vi "write byte array.vi"(8 "error in":errorcluster, 10 "specs":T1[](array[typedef]), 11 "message":variant) -> (0 "error out":errorcluster, 3 "byte array":u8[](array[numeric]))   [LabVIEW 2013, in "protocol buffers encoder.lvlib"]
uses:
  protocol buffers encoder.lvlib
  message specification.ctl
  field descriptor.ctl
  quantity.ctl
  wire type.ctl
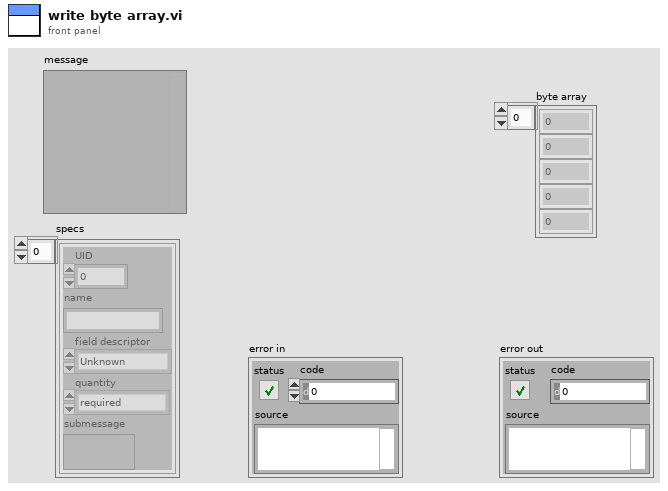
[diagram p1: front panel]
types:
  T1 = typedef "protocol buffers encoder.lvlib/message specification.ctl" = cluster{"UID":u64, "name":string, "field descriptor":T2, "quantity":T3, "submessage":variant}
  T2 = typedef "protocol buffers encoder.lvlib/field descriptor.ctl" = enum16{"Unknown", "dbl", "sgl", "i64", "u64", "i32", "fixed64", "fixed32", "bool", "string", "group", "message", "bytes", "u32", "enum", "sfixed32", "sfixed64", "sint32", "sint64"}
  T3 = typedef "protocol buffers encoder.lvlib/quantity.ctl" = enum16{"required", "optional", "repeated", "repeated/packed"}
  T4 = typedef "protocol buffers encoder.lvlib/wire type.ctl" = enum8{"Varint", "64 bit", "Length Delimited", "Start Group", "End Group", "32 bit"}
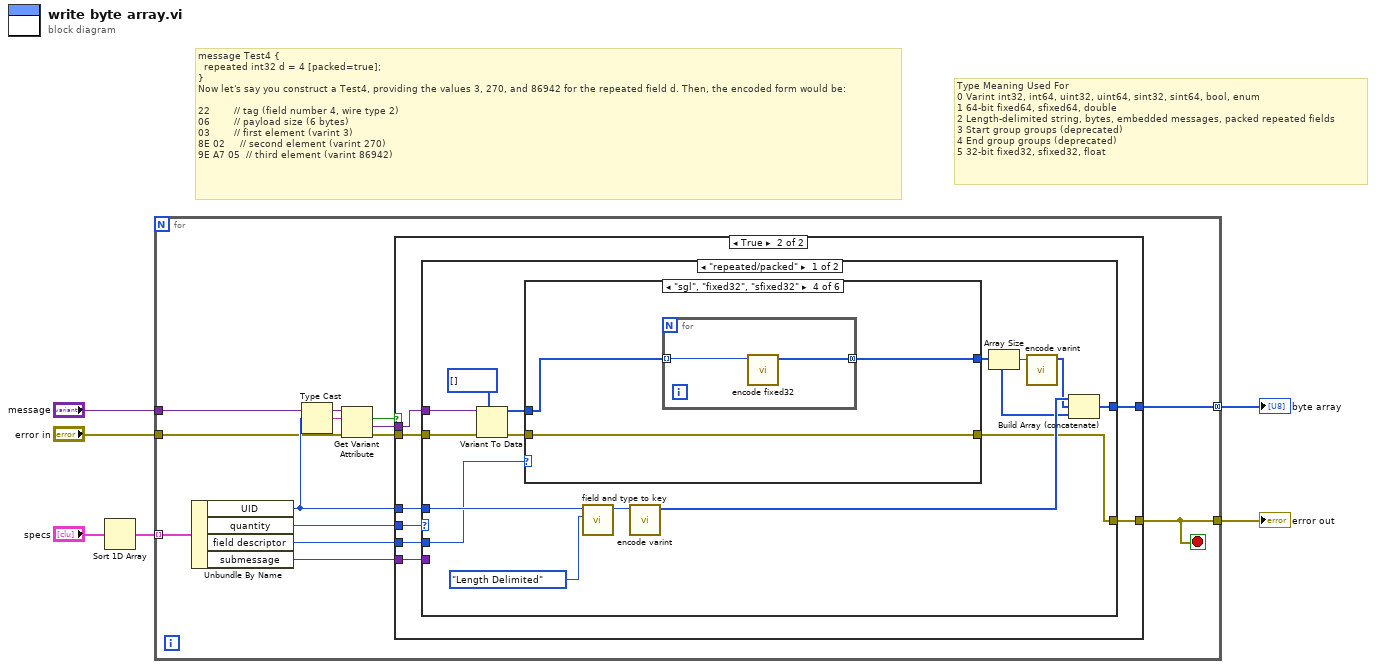
[diagram p0: block diagram]
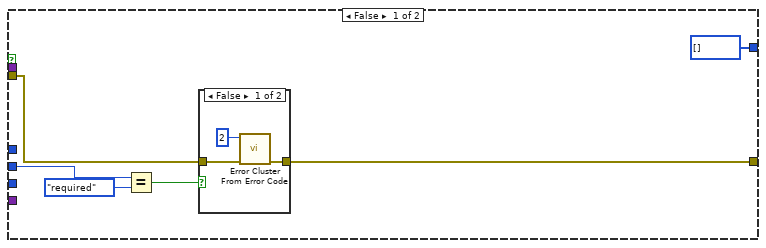
[diagram p2: hidden frame]
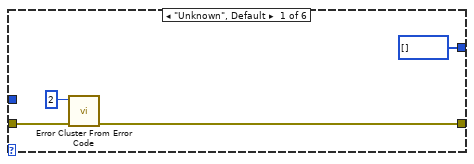
[diagram p4: hidden frame]
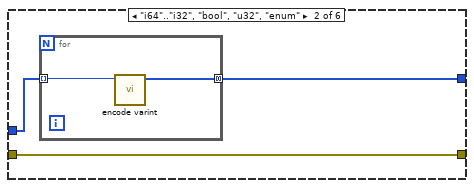
[diagram p5: hidden frame]
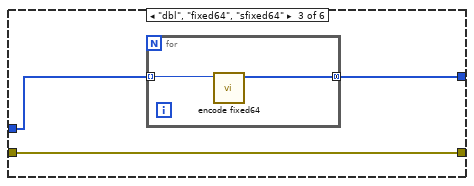
[diagram p6: hidden frame]
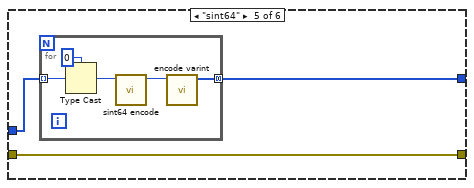
[diagram p7: hidden frame]
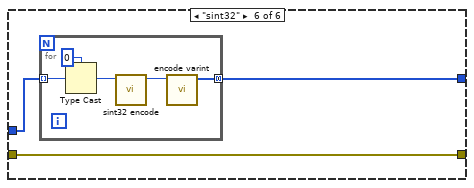
[diagram p8: hidden frame]
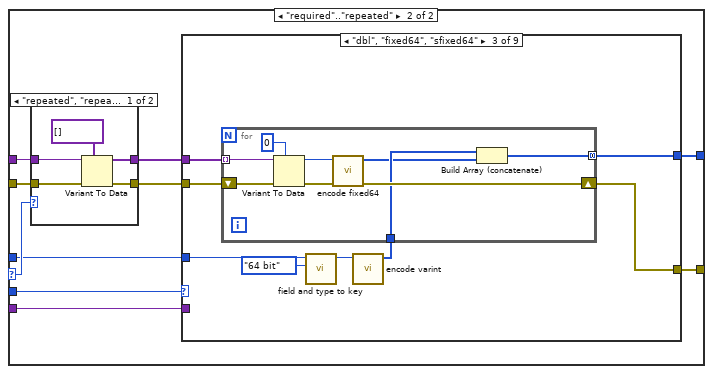
[diagram p9: hidden frame]
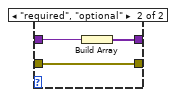
[diagram p10: hidden frame]
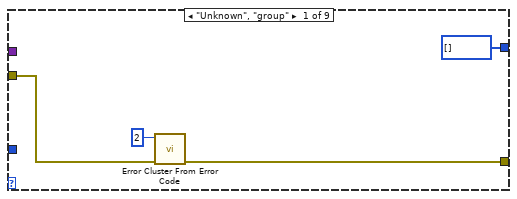
[diagram p11: hidden frame]
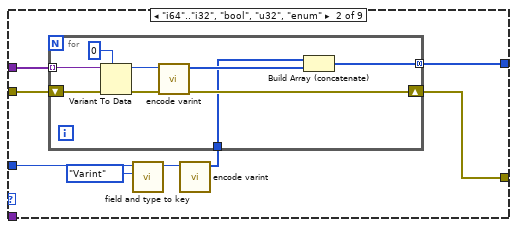
[diagram p12: hidden frame]
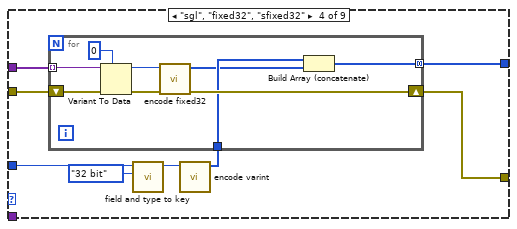
[diagram p13: hidden frame]
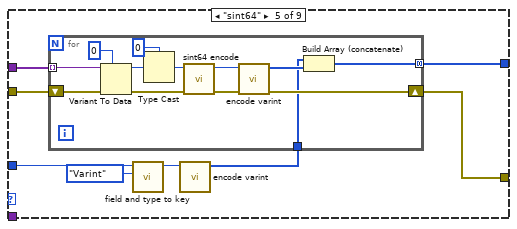
[diagram p14: hidden frame]
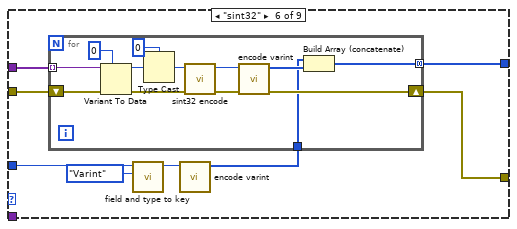
[diagram p15: hidden frame]
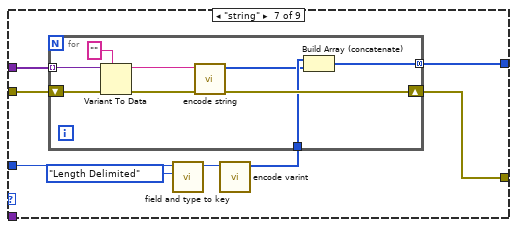
[diagram p16: hidden frame]
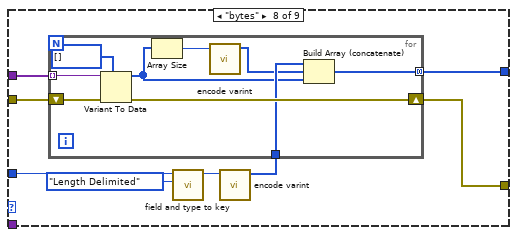
[diagram p17: hidden frame]
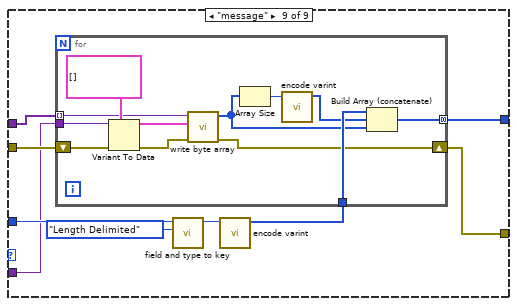
[diagram p18: hidden frame]
diagram:
  # "message Test4 {\n  repeated int32 d = 4 [packed=true];\n}\nNow let's say you construct a Test4, providing the values 3, 270, and 86942 for the repeated field d. Then, the encoded form would be:\n\n22        // tag (field number 4, wire type 2)\n06        // payload size (6 bytes)\n03        // first element (varint 3)\n8E 02     // second element (varint 270)\n9E A7 05  // third element (varint 86942)"
  # "Type\tMeaning\tUsed For\n0\tVarint\tint32, int64, uint32, uint64, sint32, sint64, bool, enum\n1\t64-bit\tfixed64, sfixed64, double\n2\tLength-delimited\tstring, bytes, embedded messages, packed repeated fields\n3\tStart group\tgroups (deprecated)\n4\tEnd group\tgroups (deprecated)\n5\t32-bit\tfixed32, sfixed32, float"
  n1 = Sort 1D Array(array="specs") -> (sorted array=w3:T1[])
  n2 = for {
    tunnel: w3 -> [w19] mode=indexing
    tunnel: "message" -> [w18]
    tunnel: [w13] -> w4
    tunnel: [w8] -> w2 mode=concatenating
    tunnel: "error in" -> [w7]
    stop <- w13 stop-if-true
    n3 = Unbundle By Name(w19) -> ("UID"=w9:u64, "quantity"=w10:T3, "field descriptor"=w12:T2, "submessage"=w11:variant)
    n4 = Type Cast(x=w9) -> (*(type *) &x=w17:string)  [unwired: 1 in]
    n5 = Get Variant Attribute(Variant=w18, name=w17, error in=w7) -> (found=w14:bool, value=w15:variant, error out=w16:errorcluster)  [unwired: 1 in, 1 out]
    n6 = case shown="True" w14 {
      tunnel: w16 -> [w22 w35]
      tunnel: w15 -> [_ w34]
      tunnel: w10 -> [w25 w32]
      tunnel: [w21 w36] -> w13
      tunnel: w12 -> [_ w37]
      tunnel: w11 -> [_ w33]
      tunnel: w9 -> [_ w31]
      tunnel: [u8[] [] w30] -> w8
      frame False {
        n7 = Equal?(x=w25, y=quantity."required") -> (x = y?=w23:bool)
        n8 = case shown="False" w23 {
          tunnel: w22 -> [w27 w29]
          tunnel: [w26 w29] -> w21
          frame False {
            n9 = call <vilib>:"Error Cluster From Error Code.vi"("error in (no error)"=w27, "error code (0)"=2) -> ("error out"=w26:errorcluster)  [unwired: 7 in]
          }
          frame True {
          }
        }
      }
      frame True {
        n10 = case shown="\"repeated/packed\"" w32 {
          selector: w32 -> [_ w90]
          tunnel: w37 -> [w44 w97]
          tunnel: [w42 w96] -> w36
          tunnel: w35 -> [w50 w95]
          tunnel: w34 -> [w51 w94]
          tunnel: w33 -> [_ w91]
          tunnel: w31 -> [w47 w89]
          tunnel: [w45 w88] -> w30
          frame "repeated/packed" {
            n11 = Variant To Data(error in=w50, type=u64[] [], Variant=w51) -> (data=w41:u64[], error out=w43:errorcluster)
            n12 = case shown="\"sgl\", \"fixed32\", \"sfixed32\"" w44 {
              tunnel: w43 -> [w55 w59 w64 w69 w74 w82]
              tunnel: [w54 w59 w64 w69 w74 w82] -> w42
              tunnel: w41 -> [_ w58 w63 w68 w73 w81]
              tunnel: [u8[] [] ("byte array out") w57 w62 w67 w72 w80] -> w38
              frame "Unknown", Default {
                n13 = call <vilib>:"Error Cluster From Error Code.vi"("error in (no error)"=w55, "error code (0)"=2) -> ("error out"=w54:errorcluster)  [unwired: 7 in]
              }
              frame "i64".."i32", "bool", "u32", "enum" {
                n14 = for {
                  tunnel: w58 -> [w61] mode=indexing
                  tunnel: [w60] -> w57 mode=concatenating
                  n15 = call "encode varint.vi"("value"=w61) -> ("byte array out"=w60:u8[])  [unwired: 10 in]
                }
              }
              frame "dbl", "fixed64", "sfixed64" {
                n16 = for {
                  tunnel: w63 -> [w66] mode=indexing
                  tunnel: [w65] -> w62 mode=concatenating
                  n17 = call "encode fixed64.vi"("U64"=w66) -> ("byte array out"=w65:u8[])  [unwired: 10 in]
                }
              }
              frame "sgl", "fixed32", "sfixed32" {
                n18 = for {
                  tunnel: w68 -> [w70] mode=indexing
                  tunnel: [w71] -> w67 mode=concatenating
                  n19 = call "encode fixed32.vi"("u32"=w70) -> ("byte array out"=w71:u8[])  [unwired: 10 in]
                }
              }
              frame "sint64" {
                n20 = for {
                  tunnel: w73 -> [w78] mode=indexing
                  tunnel: [w79] -> w72 mode=concatenating
                  n21 = Type Cast(type=i64 0, x=w78) -> (*(type *) &x=w76:i64)
                  n22 = call "sint64 encode.vi"("sint64"=w76) -> ("zigzag32"=w77:u64)  [unwired: 10 in]
                  n23 = call "encode varint.vi"("value"=w77) -> ("byte array out"=w79:u8[])  [unwired: 10 in]
                }
              }
              frame "sint32" {
                n24 = for {
                  tunnel: w81 -> [w86] mode=indexing
                  tunnel: [w87] -> w80 mode=concatenating
                  n25 = Type Cast(type=0, x=w86) -> (*(type *) &x=w84:i32)
                  n26 = call "sint32 encode.vi"("sint32"=w84) -> ("zigzag32"=w83:u32)  [unwired: 10 in]
                  n27 = call "encode varint.vi"("value"=w83) -> ("byte array out"=w87:u8[])  [unwired: 10 in]
                }
              }
            }
            n28 = call "field and type to key.vi"("wire type"=wire_type."Length Delimited", "field number"=w47) -> ("key"=w49:u64)  [unwired: 9 in]
            n29 = call "encode varint.vi"("value"=w49) -> ("byte array out"=w46:u8[])  [unwired: 10 in]
            n30 = Array Size(array=w38) -> (size(s)=w39:i32)
            n31 = call "encode varint.vi"("value"=w39) -> ("byte array out"=w40:u8[])  [unwired: 10 in]
            n32 = Build Array (concatenate)(w46, w40, w38) -> (w45:u8[])
          }
          frame "required".."repeated" {
            n33 = case shown="\"repeated\", \"repeated/packed\"" w90 {
              tunnel: w95 -> [w100 w103]
              tunnel: w94 -> [w101 w105]
              tunnel: [w99 w104] -> w93
              tunnel: [w98 w103] -> w92
              frame "repeated", "repeated/packed" {
                n34 = Variant To Data(error in=w100, type=variant[] [], Variant=w101) -> (data=w99:variant[], error out=w98:errorcluster)
              }
              frame "required", "optional" {
                n35 = Build Array(w105) -> (w104:variant[])
              }
            }
            n36 = case shown="\"dbl\", \"fixed64\", \"sfixed64\"" w97 {
              tunnel: [w108 w115 w131 w147 w163 w182 w201 w217 w235] -> w96
              tunnel: w93 -> [_ w116 w132 w148 w164 w183 w202 w218 w236]
              tunnel: w92 -> [w106 w117 w133 w149 w165 w184 w203 w219 w237]
              tunnel: w91 -> [_ _ _ _ _ _ _ _ w229]
              tunnel: w89 -> [_ w113 w129 w145 w161 w180 w199 w215 w233]
              tunnel: [u8[] [] w110 w126 w142 w158 w177 w196 w212 w230] -> w88
              frame "Unknown", "group" {
                n37 = call <vilib>:"Error Cluster From Error Code.vi"("error in (no error)"=w106, "error code (0)"=2) -> ("error out"=w108:errorcluster)  [unwired: 7 in]
              }
              frame "i64".."i32", "bool", "u32", "enum" {
                n38 = call "field and type to key.vi"("wire type"=wire_type."Varint", "field number"=w113) -> ("key"=w114:u64)  [unwired: 9 in]
                n39 = call "encode varint.vi"("value"=w114) -> ("byte array out"=w111:u8[])  [unwired: 10 in]
                n40 = for {
                  shift-right: [w122] -> w115
                  shift-left: w117 -> [w124]
                  tunnel: w116 -> [w125] mode=indexing
                  tunnel: w111 -> [w120]
                  tunnel: [w118] -> w110 mode=concatenating
                  n41 = Variant To Data(error in=w124, type=u64 0, Variant=w125) -> (data=w119:u64, error out=w122:errorcluster)
                  n42 = call "encode varint.vi"("value"=w119) -> ("byte array out"=w121:u8[])  [unwired: 10 in]
                  n43 = Build Array (concatenate)(w120, w121) -> (w118:u8[])
                }
              }
              frame "dbl", "fixed64", "sfixed64" {
                n44 = call "field and type to key.vi"("wire type"=wire_type."64 bit", "field number"=w129) -> ("key"=w130:u64)  [unwired: 9 in]
                n45 = call "encode varint.vi"("value"=w130) -> ("byte array out"=w127:u8[])  [unwired: 10 in]
                n46 = for {
                  shift-right: [w138] -> w131
                  shift-left: w133 -> [w140]
                  tunnel: w132 -> [w141] mode=indexing
                  tunnel: w127 -> [w137]
                  tunnel: [w136] -> w126 mode=concatenating
                  n47 = Variant To Data(error in=w140, type=u64 0, Variant=w141) -> (data=w135:u64, error out=w138:errorcluster)
                  n48 = call "encode fixed64.vi"("U64"=w135) -> ("byte array out"=w134:u8[])  [unwired: 10 in]
                  n49 = Build Array (concatenate)(w137, w134) -> (w136:u8[])
                }
              }
              frame "sgl", "fixed32", "sfixed32" {
                n50 = call "field and type to key.vi"("wire type"=wire_type."32 bit", "field number"=w145) -> ("key"=w146:u64)  [unwired: 9 in]
                n51 = call "encode varint.vi"("value"=w146) -> ("byte array out"=w143:u8[])  [unwired: 10 in]
                n52 = for {
                  shift-right: [w154] -> w147
                  shift-left: w149 -> [w156]
                  tunnel: w148 -> [w157] mode=indexing
                  tunnel: w143 -> [w153]
                  tunnel: [w152] -> w142 mode=concatenating
                  n53 = Variant To Data(error in=w156, type=u32 0, Variant=w157) -> (data=w150:u32, error out=w154:errorcluster)
                  n54 = call "encode fixed32.vi"("u32"=w150) -> ("byte array out"=w151:u8[])  [unwired: 10 in]
                  n55 = Build Array (concatenate)(w153, w151) -> (w152:u8[])
                }
              }
              frame "sint64" {
                n56 = call "field and type to key.vi"("wire type"=wire_type."Varint", "field number"=w161) -> ("key"=w162:u64)  [unwired: 9 in]
                n57 = call "encode varint.vi"("value"=w162) -> ("byte array out"=w159:u8[])  [unwired: 10 in]
                n58 = for {
                  shift-right: [w173] -> w163
                  shift-left: w165 -> [w175]
                  tunnel: w164 -> [w176] mode=indexing
                  tunnel: w159 -> [w171]
                  tunnel: [w170] -> w158 mode=concatenating
                  n59 = Variant To Data(error in=w175, type=u64 0, Variant=w176) -> (data=w168:u64, error out=w173:errorcluster)
                  n60 = Type Cast(type=i64 0, x=w168) -> (*(type *) &x=w166:i64)
                  n61 = call "sint64 encode.vi"("sint64"=w166) -> ("zigzag32"=w169:u64)  [unwired: 10 in]
                  n62 = call "encode varint.vi"("value"=w169) -> ("byte array out"=w172:u8[])  [unwired: 10 in]
                  n63 = Build Array (concatenate)(w171, w172) -> (w170:u8[])
                }
              }
              frame "sint32" {
                n64 = call "field and type to key.vi"("wire type"=wire_type."Varint", "field number"=w180) -> ("key"=w181:u64)  [unwired: 9 in]
                n65 = call "encode varint.vi"("value"=w181) -> ("byte array out"=w178:u8[])  [unwired: 10 in]
                n66 = for {
                  shift-right: [w192] -> w182
                  shift-left: w184 -> [w194]
                  tunnel: w183 -> [w195] mode=indexing
                  tunnel: w178 -> [w190]
                  tunnel: [w189] -> w177 mode=concatenating
                  n67 = Variant To Data(error in=w194, type=u64 0, Variant=w195) -> (data=w188:u64, error out=w192:errorcluster)
                  n68 = Type Cast(type=0, x=w188) -> (*(type *) &x=w186:i32)
                  n69 = call "sint32 encode.vi"("sint32"=w186) -> ("zigzag32"=w185:u32)  [unwired: 10 in]
                  n70 = call "encode varint.vi"("value"=w185) -> ("byte array out"=w191:u8[])  [unwired: 10 in]
                  n71 = Build Array (concatenate)(w190, w191) -> (w189:u8[])
                }
              }
              frame "string" {
                n72 = call "field and type to key.vi"("wire type"=wire_type."Length Delimited", "field number"=w199) -> ("key"=w200:u64)  [unwired: 9 in]
                n73 = call "encode varint.vi"("value"=w200) -> ("byte array out"=w197:u8[])  [unwired: 10 in]
                n74 = for {
                  shift-right: [w208] -> w201
                  shift-left: w203 -> [w210]
                  tunnel: w202 -> [w211] mode=indexing
                  tunnel: w197 -> [w207]
                  tunnel: [w206] -> w196 mode=concatenating
                  n75 = Variant To Data(error in=w210, type="", Variant=w211) -> (data=w205:string, error out=w208:errorcluster)
                  n76 = call "encode string.vi"("String"=w205) -> ("byte array out"=w204:u8[])  [unwired: 10 in]
                  n77 = Build Array (concatenate)(w207, w204) -> (w206:u8[])
                }
              }
              frame "bytes" {
                n78 = call "field and type to key.vi"("wire type"=wire_type."Length Delimited", "field number"=w215) -> ("key"=w216:u64)  [unwired: 9 in]
                n79 = call "encode varint.vi"("value"=w216) -> ("byte array out"=w213:u8[])  [unwired: 10 in]
                n80 = for {
                  shift-right: [w226] -> w217
                  shift-left: w219 -> [w227]
                  tunnel: w218 -> [w228] mode=indexing
                  tunnel: w213 -> [w225]
                  tunnel: [w224] -> w212 mode=concatenating
                  n81 = Variant To Data(error in=w227, type=u8[] [], Variant=w228) -> (data=w222:u8[], error out=w226:errorcluster)
                  n82 = Array Size(array=w222) -> (size(s)=w221:i32)
                  n83 = call "encode varint.vi"("value"=w221) -> ("byte array out"=w220:u8[])  [unwired: 10 in]
                  n84 = Build Array (concatenate)(w225, w220, w222) -> (w224:u8[])
                }
              }
              frame "message" {
                n85 = call "field and type to key.vi"("wire type"=wire_type."Length Delimited", "field number"=w233) -> ("key"=w234:u64)  [unwired: 9 in]
                n86 = call "encode varint.vi"("value"=w234) -> ("byte array out"=w231:u8[])  [unwired: 10 in]
                n87 = for {
                  shift-right: [w239] -> w235
                  shift-left: w237 -> [w245]
                  tunnel: w236 -> [w242] mode=indexing
                  tunnel: w231 -> [w249]
                  tunnel: [w248] -> w230 mode=concatenating
                  tunnel: w229 -> [w244]
                  n88 = Variant To Data(error in=w245, type=T1[] [] ("specs"), Variant=w244) -> (data=w241:T1[], error out=w240:errorcluster)
                  n89 = call "write byte array.vi"("error in"=w240, "specs"=w241, "message"=w242) -> ("error out"=w239:errorcluster, "byte array"=w238:u8[])  [unwired: 7 in]
                  n90 = Array Size(array=w238) -> (size(s)=w247:i32)
                  n91 = call "encode varint.vi"("value"=w247) -> ("byte array out"=w246:u8[])  [unwired: 10 in]
                  n92 = Build Array (concatenate)(w249, w246, w238) -> (w248:u8[])
                }
              }
            }
          }
        }
      }
    }
  }
  "byte array" <- w2
  "error out" <- w4
